vi "komendy.vi"(4 "?":bool, 5 "ILOŒÆ D¯ULI":dbl, 6 "?":bool, 7 "?":bool, 8 "KONTRAST 3":dbl, 9 "?":bool, 10 "KONTRAST in":dbl(knob) scale=0.0..1000.0, 11 "VISA Refnum in":refnum<visa-resource-name>) -> (2 "KONTRAST out":dbl, 3 "VISA Refnum out":refnum<visa-resource-name>)   [LabVIEW 2025]
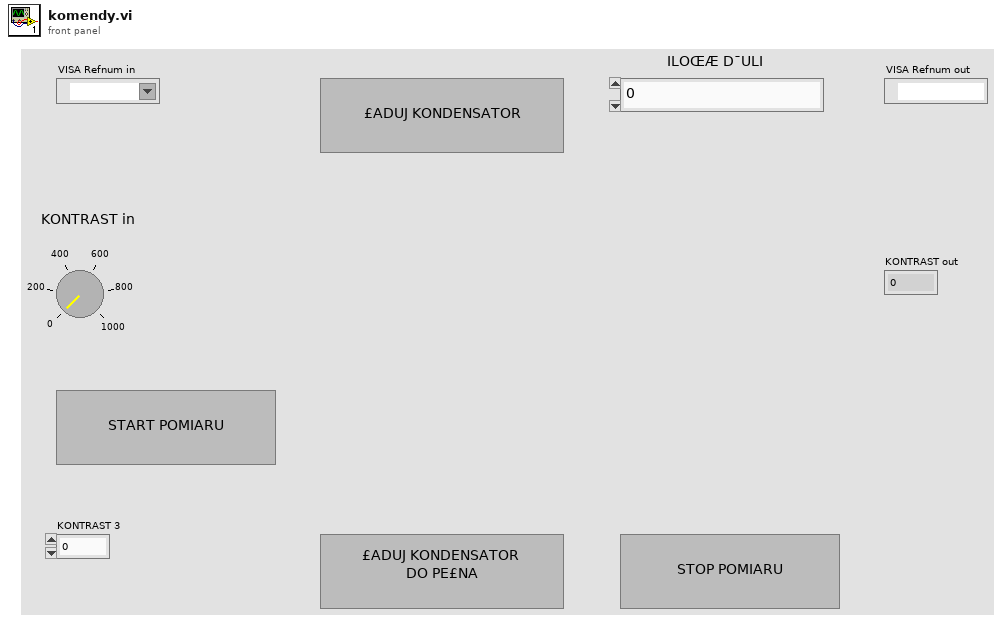
[diagram p1: front panel]
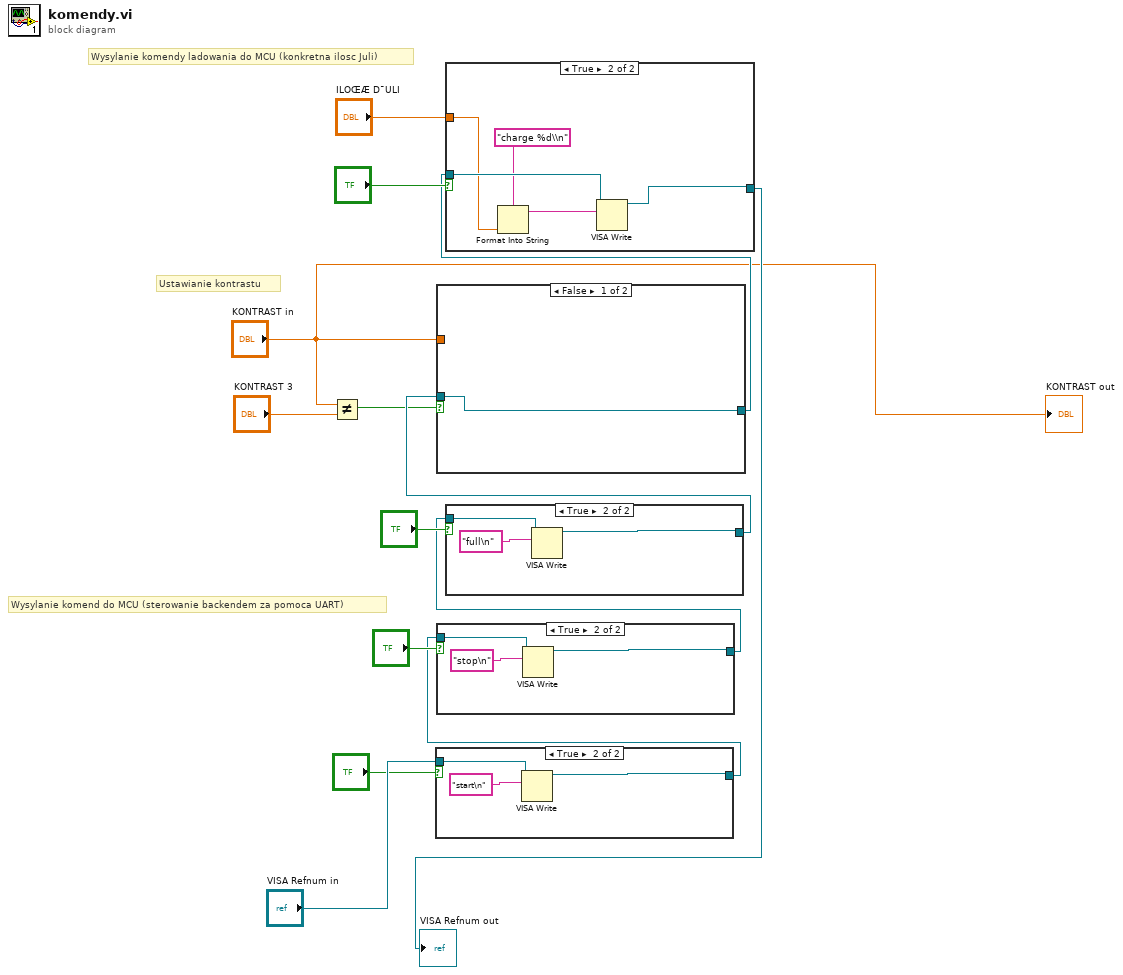
[diagram p0: block diagram]
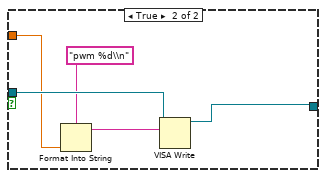
[diagram p3: hidden frame]
diagram:
  # "Wysylanie komend do MCU (sterowanie backendem za pomoca UART)"
  # "Wysylanie komendy ladowania do MCU (konkretna ilosc Juli)"
  # "Ustawianie kontrastu"
  n1 = Not Equal?(x="KONTRAST in", y="KONTRAST 3") -> (x != y?=w6:bool)
  n2 = case shown="True" "?" {
    tunnel: "VISA Refnum in" -> [w15 w18]
    tunnel: [w15 w16] -> w2
    frame False {
    }
    frame True {
      n3 = VISA Write(VISA resource name=w18, write buffer="start\n") -> (VISA resource name out=w16:refnum<visa-resource-name>)  [unwired: 1 in, 2 out]
    }
  }
  n4 = case shown="True" "?" {
    tunnel: w2 -> [w19 w22]
    tunnel: [w19 w20] -> w4
    frame False {
    }
    frame True {
      n5 = VISA Write(VISA resource name=w22, write buffer="stop\n") -> (VISA resource name out=w20:refnum<visa-resource-name>)  [unwired: 1 in, 2 out]
    }
  }
  n6 = case shown="True" "?" {
    tunnel: w4 -> [w23 w26]
    tunnel: [w23 w24] -> w7
    frame False {
    }
    frame True {
      n7 = VISA Write(VISA resource name=w26, write buffer="full\n") -> (VISA resource name out=w24:refnum<visa-resource-name>)  [unwired: 1 in, 2 out]
    }
  }
  n8 = case shown="False" w6 {
    tunnel: w7 -> [w27 w32]
    tunnel: [w27 w31] -> w12
    tunnel: "KONTRAST in" -> [_ w29]
    frame False {
    }
    frame True {
      n9 = Format Into String(format string="pwm %d\\n", w29) -> (resulting string=w30:string)  [unwired: 2 in, 1 out]
      n10 = VISA Write(VISA resource name=w32, write buffer=w30) -> (VISA resource name out=w31:refnum<visa-resource-name>)  [unwired: 1 in, 2 out]
    }
  }
  n11 = case shown="True" "?" {
    tunnel: w12 -> [w33 w38]
    tunnel: [w33 w37] -> w11
    tunnel: "ILOŒÆ D¯ULI" -> [_ w35]
    frame False {
    }
    frame True {
      n12 = Format Into String(format string="charge %d\\n", w35) -> (resulting string=w36:string)  [unwired: 2 in, 1 out]
      n13 = VISA Write(VISA resource name=w38, write buffer=w36) -> (VISA resource name out=w37:refnum<visa-resource-name>)  [unwired: 1 in, 2 out]
    }
  }
  "VISA Refnum out" <- w11
  "KONTRAST out" <- "KONTRAST in"
